vi "CRYGet Sound Device Informaion.vi"(8 "error in (no error)":errorcluster, 10 "isInput?":bool, 11 "device":u32) -> (0 "error out":errorcluster, 2 "Capabilities":T1, 3 "Device Name":string)   [LabVIEW 2013]
uses:
  CRYSound.dll
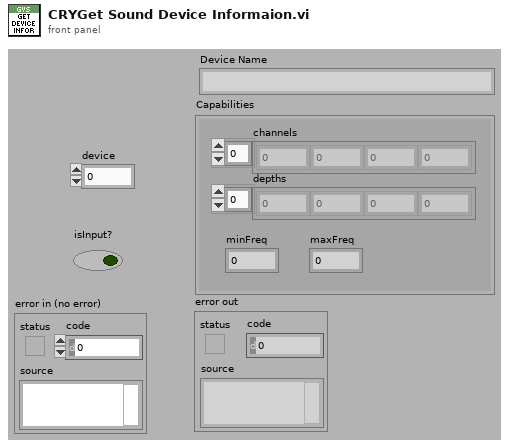
[diagram p1: front panel]
types:
  T1 = cluster{"channels":i32[], "depths":i32[], "minFreq":dbl, "maxFreq":dbl}
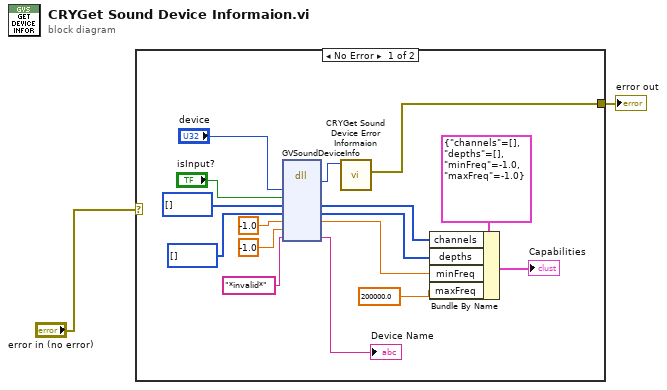
[diagram p0: block diagram]
diagram:
  n1 = case shown="No Error" "error in (no error)" {
    selector: "error in (no error)" -> [_ w19]
    tunnel: [w12 w19] -> w2
    frame No Error {
      n2 = dll-call lib="D:/LabView_Project/CRY6181/CRYSound.dll" fn="GVSoundDeviceInfo"("device"="device", "isInput"="isInput?", "channels"=i32[] [] ("numChannels"), "depths"=i32[] [] ("sampleDepths"), "minFreq"=-1.0, "maxFreq"=-1.0, "devName"="*invalid*") -> ("return type"=w13:i32, "channels"=w7:i32[], "depths"=w8:i32[], "minFreq"=w9:dbl, "devName"=→"Device Name":string)  [unwired: 5 in, 3 out]
      n3 = call "CRYGet Sound Device Error Informaion.vi"("Error Code"=w13) -> ("error out"=w12:errorcluster)  [unwired: 10 out]
      n4 = Bundle By Name(cluster=T1 {"channels"=[], "depths"=[], "minFreq"=-1.0, "maxFreq"=-1.0} ("Capabilities"), "channels"=w7, "depths"=w8, "minFreq"=w9, "maxFreq"=200000.0) -> (→"Capabilities":T1)
    }
    frame Error {
    }
  }
  "error out" <- w2
